vi "CRYProject Editor PIC ReadWrite Project Log.vi"(9 "sData":string, 11 "sAction":string) -> (1 "sDataList_Out":string[](array[string]), 2 "sData_Out":string)   [LabVIEW 2013]
uses:
  CRYMainGlobal.vi
  CRYProject Editor Global.vi
  CRYSystem/Misc/SubVI/CRYMisc vis settings global.vi
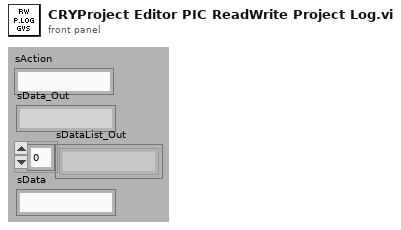
[diagram p1: front panel]
types:
  T1 = typedef "CRYTS.ctl" = cluster{"No.TS":u16, "TS File Path":path, "TS Name":string, "EditStepName":string, "Steps":T2[], "New State":bool, "Change State":bool, "Flattened CurveLib Data":string, "Document Data":string, "EditStepNo":u16, "Operator Start File":string, "Sequence Type":string, "Sequence Language":string}
  T2 = typedef "CRYStep.ctl" = cluster{"No.VI":i32, "Category":string, "StepName":string, "Seq setup flattened":string, "Comment":string, "Steps config.":bool[], "Jump config":i32[], "Start":dbl, "Increment":dbl, "Name":string, "Unit":string, "Y data":u16, "Y prefix":string, "Y dB ref":dbl, "Y unit":string, "Repeat State Array":cluster{"Start":dbl, "Increment":dbl, "Count":i32, "Num":i32}[]}
  T3 = cluster{"EventName":string, "Arg1":string, "Numeric":u16, "Numeric 2":u16, "AddSteps ":refnum<vi>, "Arg1 2":string, "Arg1 3":string, "Boolean":bool}
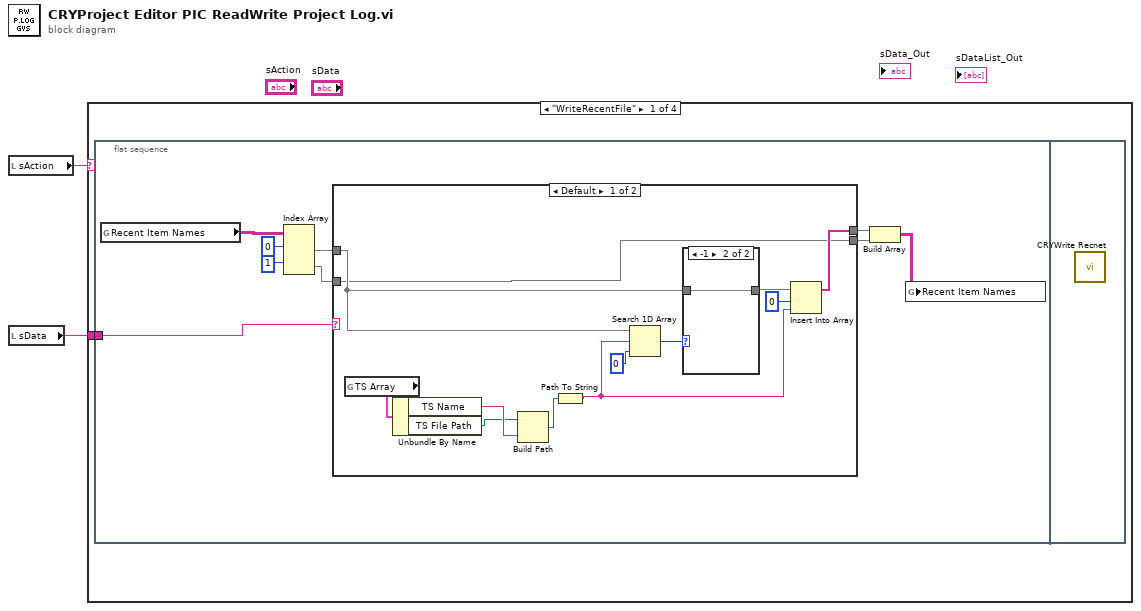
[diagram p0: block diagram]
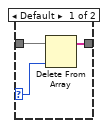
[diagram p2: hidden frame]
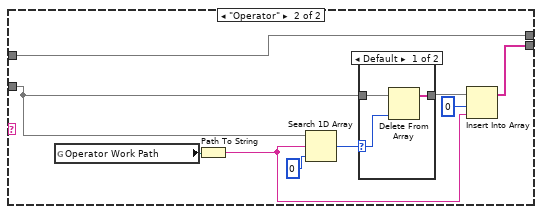
[diagram p3: hidden frame]
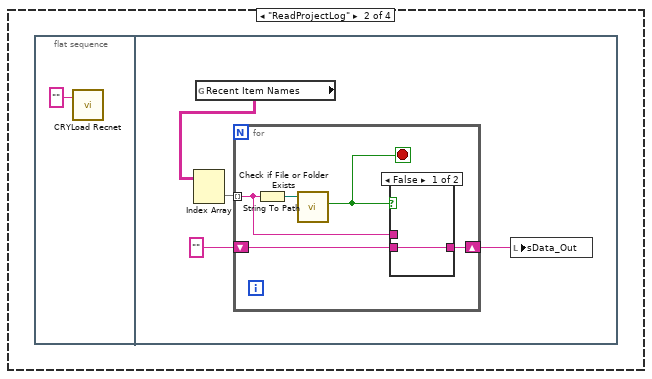
[diagram p5: hidden frame]
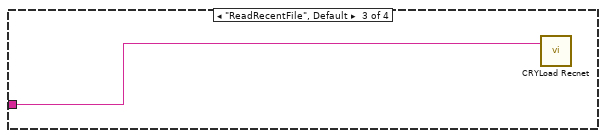
[diagram p7: hidden frame]
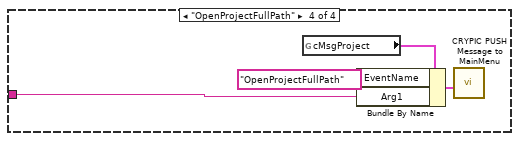
[diagram p8: hidden frame]
diagram:
  n1 = local read "sAction"() -> (w2:string)
  n2 = local read "sData"() -> (w1:string)
  n3 = case shown="\"WriteRecentFile\"" w2 {
    tunnel: w1 -> [w3 _ w54 w58]
    frame "WriteRecentFile" {
      n4 = flat-sequence {
        tunnel: w3 -> [w12]
        frame #0 {
          n5 = global read "CRYMainGlobal.vi" "Recent Item Names"() -> (w8:string[][])
          n6 = Index Array(array=w8, index (row) #1=0 ("disabled index (col)"), index (row) #2=1 ("index (row)")) -> (element #1=w5:string[], element #2=w4:string[])  [unwired: 2 in]
          n7 = case shown="Default" w12 {
            tunnel: [w19 w30] -> w10
            tunnel: [w17 w31] -> w9
            tunnel: w5 -> [w18 w30]
            tunnel: w4 -> [w17 w29]
            frame Default {
              n8 = global read "CRYProject Editor Global.vi" "TS Array"() -> (w24:T1)
              n9 = Unbundle By Name(w24) -> ("TS Name"=w16:string, "TS File Path"=w15:path)
              n10 = Build Path(base path=w15, name or relative path=w16) -> (appended path=w13:path)
              n11 = Path To String(path=w13) -> (string=w14:string)
              n12 = Search 1D Array(1D array=w18, element=w14, start index (0)=0) -> (index of element=w22:i32)
              n13 = case shown="-1" w22 {
                selector: w22 -> [w26 _]
                tunnel: w18 -> [w27 w28]
                tunnel: [w25 w28] -> w21
                frame Default {
                  n14 = Delete From Array(array=w27, index=w26) -> (array with subset deleted=w25:string[])  [unwired: 1 in, 1 out]
                }
                frame -1 {
                }
              }
              n15 = Insert Into Array(array=w21, index=0, new element=w14) -> (w19:string[])
            }
            frame "Operator" {
              n16 = global read "CRYMisc vis settings global.vi" "Operator Work Path"() -> (w33:path)
              n17 = Path To String(path=w33) -> (string=w32:string)
              n18 = Search 1D Array(1D array=w29, element=w32, start index (0)=0) -> (index of element=w36:i32)
              n19 = case shown="Default" w36 {
                selector: w36 -> [w39 _]
                tunnel: w29 -> [w40 w41]
                tunnel: [w38 w41] -> w35
                frame Default {
                  n20 = Delete From Array(array=w40, index=w39) -> (array with subset deleted=w38:string[])  [unwired: 1 in, 1 out]
                }
                frame -1 {
                }
              }
              n21 = Insert Into Array(array=w35, index=0, new element=w32) -> (w31:string[])
            }
          }
          n22 = Build Array(w10, w9) -> (w11:string[][])
          n23 = global write "CRYMainGlobal.vi" "Recent Item Names"(w11) -> ()
        }
        frame #1 {
          n24 = call "CRYWrite Recnet.vi"() -> ()  [unwired: 3 in]
        }
      }
    }
    frame "ReadProjectLog" {
      n25 = flat-sequence {
        frame #0 {
          n26 = call "CRYLoad Recnet.vi"("menu tag"="") -> ()  [unwired: 1 in, 1 out]
        }
        frame #1 {
          n27 = global read "CRYMainGlobal.vi" "Recent Item Names"() -> (w46:string[][])
          n28 = Index Array(array=w46) -> (element=w45:string[])  [unwired: 2 in]
          n29 = for {
            tunnel: w45 -> [w49] mode=indexing
            shift-right: [w48] -> w43
            shift-left: "" -> [w50]
            stop <- w47 stop-if-true
            n30 = String To Path(string=w49) -> (path=w51:path)
            n31 = call <vilib>:"Check if File or Folder Exists.vi"("path"=w51) -> ("file or folder exists?"=w47:bool)  [unwired: 8 in, 2 out]
            n32 = case shown="False" w47 {
              tunnel: w50 -> [w52 _]
              tunnel: w49 -> [_ w53]
              tunnel: [w52 w53] -> w48
              frame False {
              }
              frame True {
              }
            }
          }
          n33 = local write "sData_Out"(w43) -> ()
        }
      }
    }
    frame "ReadRecentFile", Default {
      n34 = call "CRYLoad Recnet.vi"("menu tag"=w54) -> ()  [unwired: 1 in, 1 out]
    }
    frame "OpenProjectFullPath" {
      n35 = global read "CRYProject Editor Global.vi" "cMsgProject"() -> (w57:T3)
      n36 = Bundle By Name(cluster=w57, "EventName"="OpenProjectFullPath", "Arg1"=w58) -> (w55:T3)
      n37 = call "CRYPIC PUSH Message to MainMenu.vi"("cMsgProject"=w55) -> ()  [unwired: 11 in]
    }
  }
